vi "Create AO waveforms _lockin reference_2.vi"(9 "sampling info":cluster{"Fs":dbl, "#s":dbl}={"Fs"=1000.0, "#s"=1000.0} {"Fs" format="%.2p"}, 10 "reset signal":bool, 11 "Lockin":T1={"REF f (Hz)"=[13.0, 13.0, 13.0, 13.0, 13.0, 13.0, 13.0, 13.0], "REF phi (deg)"=[0.0, 0.0, 0.0, 0.0, 0.0, 0.0, 0.0, 0.0]} {"REF phi (deg)" format="%#_3g"}) -> (0 "phase out":dbl[](array[numeric]), 1 "AO Array":waveform(dbl)[](array[waveform]), 3 "Lockin 2":T1={"REF f (Hz)"=[13.0, 13.0, 13.0, 13.0, 13.0, 13.0, 13.0, 13.0], "REF phi (deg)"=[0.0, 0.0, 0.0, 0.0, 0.0, 0.0, 0.0, 0.0]} {"REF phi (deg)" format="%#_3g"})   [LabVIEW 2013]
uses:
  <vilib>/measure/NI_MABase.lvlib
panel:
  out "Waveform Graph 2":waveform(dbl)[](graph)=[{"t0"=timestamp(0 s since 1904-01-01), "dt"=4.8828125e-06, "Y"=array[20480 elements]}, {"t0"=timestamp(0 s since 1904-01-01), "dt"=4.8828125e-06, "Y"=array[20480 elements]}, {"t0"=timestamp(0 s since 1904-01-01), "dt"=4.8828125e-06, "Y"=array[20480 elements]}, {"t0"=timestamp(0 s since 1904-01-01), "dt"=4.8828125e-06, "Y"=array[20480 elements]}, {"t0"=timestamp(0 s since 1904-01-01), "dt"=4.8828125e-06, "Y"=array[20480 elements]}, {"t0"=timestamp(0 s since 1904-01-01), "dt"=4.8828125e-06, "Y"=array[20480 elements]}, {"t0"=timestamp(0 s since 1904-01-01), "dt"=4.8828125e-06, "Y"=array[20480 elements]}, {"t0"=timestamp(0 s since 1904-01-01), "dt"=4.8828125e-06, "Y"=array[20480 elements]}]
  out "Numeric":i32
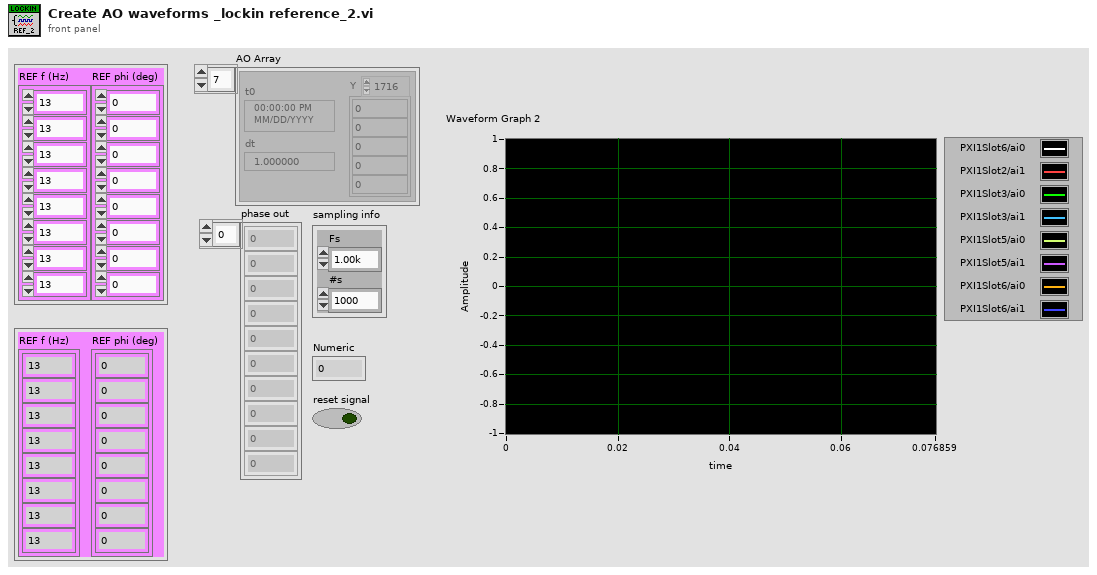
[diagram p1: front panel]
types:
  T1 = cluster{"REF f (Hz)":dbl[], "REF phi (deg)":dbl[]}
  T2 = enum16{"Sine Wave", "Triangle Wave", "Square Wave", "Sawtooth Wave"}
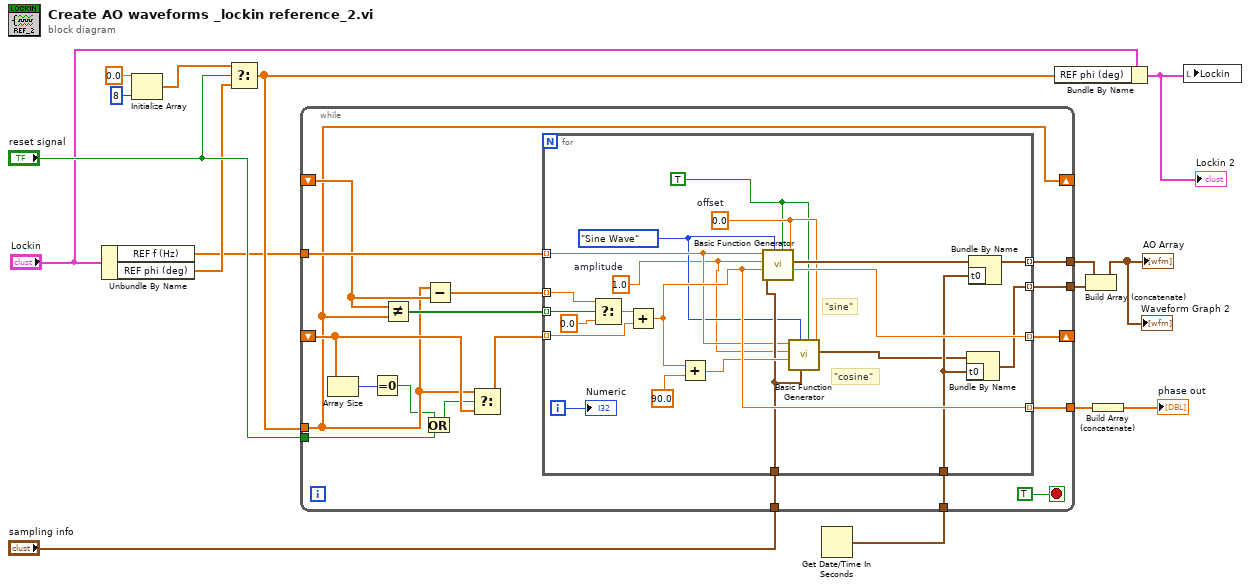
[diagram p0: block diagram]
diagram:
  n1 = Unbundle By Name("Lockin") -> ("REF f (Hz)"=w4:dbl[], "REF phi (deg)"=w5:dbl[])
  n2 = Initialize Array(0.0 ("element"), 8 ("dimension size")) -> (w12:dbl[])
  n3 = Select(t=w12, s="reset signal", f=w5) -> (s? t:f=w11:dbl[])
  n4 = Get Date/Time In Seconds() -> (seconds since 1Jan1904=w13:timestamp)
  n5 = while {
    tunnel: "sampling info" -> [w34]
    tunnel: [w33] -> w6
    tunnel: w11 -> [w22]
    tunnel: w4 -> [w32]
    shift-right: [w22] -> _
    shift-left: _ -> [w29]
    shift-right: [w27] -> _
    shift-left: _ -> [w24]
    tunnel: w13 -> [w25]
    tunnel: "reset signal" -> [w19]
    tunnel: [w18] -> w9
    tunnel: [w17] -> w7
    stop <- TRUE stop-if-true
    n6 = Array Size(array=w24) -> (size(s)=w23:i32)
    n7 = Equal To 0?(x=w23) -> (x = 0?=w20:bool)
    n8 = Not Equal?(x=w29, y=w22) -> (x != y?=w30:bool[])
    n9 = Or(x=w20, y=w19) -> (x .or. y?=w21:bool)
    n10 = Subtract(x=w22, y=w29) -> (x-y=w28:dbl[])
    n11 = Select(t=w22, s=w21, f=w24) -> (s? t:f=w26:dbl[])
    n12 = for {
      tunnel: w32 -> [w42] mode=indexing
      tunnel: [w54] -> w33 mode=indexing
      tunnel: w34 -> [w43]
      tunnel: w30 -> [w48] mode=indexing
      tunnel: w28 -> [w50] mode=indexing
      tunnel: [w46] -> w27 mode=indexing
      tunnel: w26 -> [w51] mode=indexing
      tunnel: w25 -> [w41]
      tunnel: [w45] -> w18 mode=indexing
      tunnel: [w39] -> w17 mode=indexing
      i -> [w47]
      w35 = TRUE ("reset signal")
      w37 = 0.0  # offset
      w38 = T2."Sine Wave" ("signal type")
      w36 = 1.0  # amplitude
      # "\"cosine\""
      # "\"sine\""
      n13 = Select(t=w50, s=w48, f=0.0) -> (s? t:f=w52:dbl)
      n14 = Add(x=w52, y=w51) -> (x+y=w45:dbl)
      n15 = Add(x=w45, y=90.0) -> (x+y=w44:dbl)
      n16 = call <vilib>:"Basic Function Generator.vi"("offset"=w37, "reset signal"=w35, "sampling info"=w43, "signal type"=w38, "phase"=w45, "amplitude"=w36, "frequency"=w42) -> ("phase out"=w46:dbl, "signal out"=w55:waveform(dbl))  [unwired: 2 in, 1 out]
      n17 = call <vilib>:"Basic Function Generator.vi"("offset"=w37, "reset signal"=w35, "sampling info"=w43, "signal type"=w38, "phase"=w44, "amplitude"=w36, "frequency"=w42) -> ("signal out"=w40:waveform(dbl))  [unwired: 2 in, 2 out]
      n18 = Bundle By Name(cluster=w40, "t0"=w41) -> (w39:waveform(dbl))
      n19 = Bundle By Name(cluster=w55, "t0"=w41) -> (w54:waveform(dbl))
      "Numeric" <- w47
    }
  }
  n20 = Bundle By Name(cluster="Lockin", "REF phi (deg)"=w11) -> (w2:T1)
  "Lockin 2" <- w2
  n21 = Build Array (concatenate)(w6, w7) -> (→"AO Array" →"Waveform Graph 2":waveform(dbl)[])
  n22 = Build Array (concatenate)(w9) -> (→"phase out":dbl[])
  n23 = local write "Lockin"(w2) -> ()
